vi "Event Handle Loop_Add Button.vi"(8 "error in (no error)":errorcluster, 10 "Button Attribute []":T1[](array[typedef]), 11 "QMenu Class in":refnum<class "QMenu Class.lvclass">) -> (0 "error out":errorcluster, 3 "QMenu Class out":refnum<class "QMenu Class.lvclass">)   [LabVIEW 2020, in "QTab.lvlib" / "QMenu Class.lvclass"]
uses:
  QMenu Class.lvclass
  Button Attribute.ctl
  QMenu Class.lvclass/QMenu Class.ctl
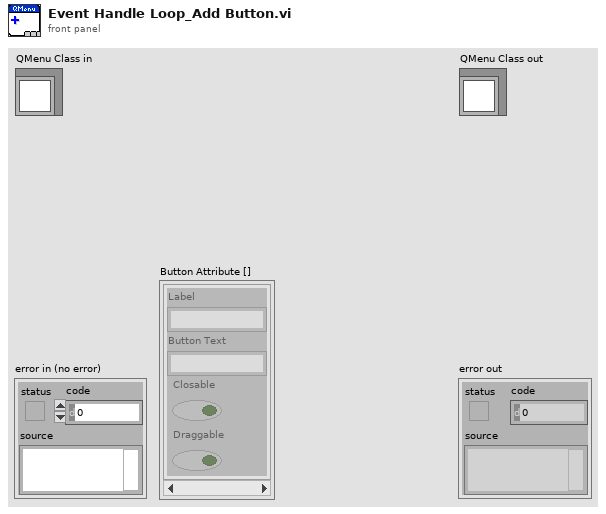
[diagram p1: front panel]
types:
  T1 = typedef "QTab.lvlib/QMenu Class.lvclass/Button Attribute.ctl" = cluster{"Label":string, "Button Text":string, "Closable":bool, "Draggable":bool}
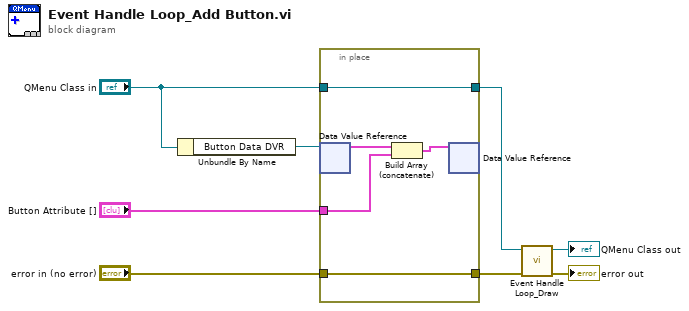
[diagram p0: block diagram]
diagram:
  n1 = Unbundle By Name("QMenu Class in") -> ("Button Data DVR"=w8:refnum<data-value>)
  n2 = in-place {
    in-place-border: "QMenu Class in" -> [w13]
    in-place-border: [w13] -> w3
    in-place-border: "error in (no error)" -> [w12]
    in-place-border: [w12] -> w4
    in-place-border: "Button Attribute []" -> [w10]
    n3 = in-place-dvr #1(w8) -> (w11:T1[])  [unwired: 1 out]
    n4 = Build Array (concatenate)(w11, w10) -> (w9:T1[])
    n5 = in-place-dvr #1(w9) -> ()  [unwired: 2 out]
  }
  n6 = call "Event Handle Loop_Draw.vi"("error in (no error)"=w4, "QMenu Class in"=w3) -> ("error out"=→"error out":errorcluster, "QMenu Class out"=→"QMenu Class out":refnum<class "QMenu Class.lvclass">)  [unwired: 8 in]
